vi "GetStoredImage.vi"(0 "reference in":refnum<class "LcPictureBox.lvclass">, 2 "ImageName":string, 5 "error in (no error)":errorcluster) -> (14 "reference out":refnum<class "LcPictureBox.lvclass">, 15 "ImageOut":refnum<k24>, 17 "ImageSize":cluster{"Width":i32, "Height":i32}, 19 "error out":errorcluster)   [LabVIEW 2020, in "LcPictureBox.lvclass"]
uses:
  LcPictureBox.lvclass
  System.Drawing
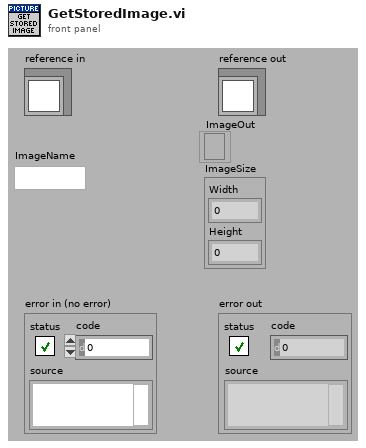
[diagram p1: front panel]
types:
  T1 = typedef "LcPictureBox.lvclass/ObjectAttributes.ctl" = cluster{"PictureBox":refnum<k24>, "ImageSize":cluster{"Width":i32, "Height":i32}, "PenMemory":map{cluster{"Alpha(100%)":dbl, "Color(Black)":u32, "Pen(Width=1, Solid)":T2}, refnum<k24>}, "GraphicsRef":refnum<k24>, "BrushMemory":map{cluster{"Alpha(100%)":dbl, "Color(Black)":u32}, refnum<k24>}, "Images":refnum<k24>[], "ImageIndex":i32, "BgColor(None)":u32, "LoadedImages":map{string, cluster{"ImageOut":refnum<k24>, "ImageSize":cluster{"Width":i32, "Height":i32}}}, "ColorsMemory":map{cluster{"Alpha(100%)":dbl, "Color(Black)":u32}, refnum<k24>}, "CacheSize":i32, "PictureBoxActiveXReference":refnum<vi>, "Scale":sgl, "Offset":cluster{"x":sgl, "y":sgl}, "zoom_center":cluster{"X":i32, "Y":i32}, "ImagesCreated":refnum<k24>[]}
  T2 = typedef "LcPictureBox.lvclass/Pen.ctl" = cluster{"Width":u16, "Style":enum32{"Solid", "Dash", "Dot", "DashDot", "DashDotDot"}}
  T3 = map{string, cluster{"ImageOut":refnum<k24>, "ImageSize":cluster{"Width":i32, "Height":i32}}}
  T4 = cluster{"ImageOut":refnum<k24>, "ImageSize":cluster{"Width":i32, "Height":i32}}
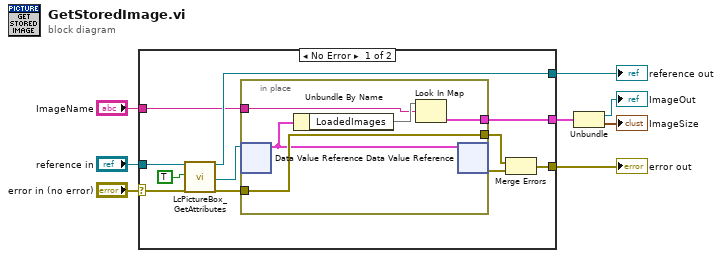
[diagram p0: block diagram]
diagram:
  n1 = case shown="No Error" "error in (no error)" {
    selector: "error in (no error)" -> [w14 w26]
    tunnel: [w18 w26] -> w7
    tunnel: [w16 w25] -> w5
    tunnel: "reference in" -> [w17 w25]
    tunnel: "ImageName" -> [w9 _]
    tunnel: [w10 _] -> w3
    frame No Error {
      n2 = call "LcPictureBox_GetAttributes.vi"("reference in"=w17, "OnlyGetDvrReference(False)"=TRUE, "error in (no error)"=w14) -> ("reference out"=w16:refnum<class "LcPictureBox.lvclass">, "DataRef"=w15:refnum<data-value>, "error out"=w13:errorcluster)  [unwired: 13 in, 1 out]
      n3 = in-place {
        in-place-border: w13 -> [w24]
        in-place-border: [w24] -> w12
        in-place-border: w9 -> [w21]
        in-place-border: [w20] -> w10
        n4 = in-place-dvr #1(w15) -> (w23:T1)  [unwired: 1 out]
        n5 = Unbundle By Name(w23) -> ("LoadedImages"=w22:T3)
        n6 = Look In Map(map=w22, key=w21) -> (value=w20:T4)  [unwired: 1 in, 1 out]
        n7 = in-place-dvr #1(w23) -> (w19:errorcluster)  [unwired: 1 out]
      }
      n8 = Merge Errors(w12, w19) -> (w18:errorcluster)
    }
    frame Error {
    }
  }
  "error out" <- w7
  "reference out" <- w5
  n9 = Unbundle(w3) -> ("ImageOut"=→"ImageOut":refnum<k24>, "ImageSize"=→"ImageSize":cluster{"Width":i32, "Height":i32})
